vi "Fetch Rx Data (I16 multi).vi"(0 "Register Bus":T1, 2 "vertical range [Vpp]":dbl=2.0 format="%#_6p", 5 "number of samples":u32=8196, 9 "timeout [s]":dbl=10.0, 11 "error in":errorcluster, 13 "leading samples to trim":i32) -> (3 "scaling (V/code)":dbl, 4 "Register Bus (out)":T1, 6 "I":i16[](array[numeric]), 8 "Q":i16[](array[numeric]), 15 "error out":errorcluster)   [LabVIEW 2017]
doc: "Fetch Rx data from the device. It's required to call <b>Configure Stream</b> and <b>Initiate Stream</b> before calling this VI."
uses:
  <instrlib>/_niInstr/Register Bus/v0/Host/Public/Register Bus Session.ctl
  <instrlib>/_niInstr/Register Bus/v0/Host/Private/Session Data.ctl
  Rx FPGA VI Reference.ctl
  <vilib>/rvi/errors/niLvFpgaAdjustHostInterfaceError.vi
  <vilib>/rvi/interface/nirviMethod/nirviMethod.xnode
  <instrlib>/_niInstr/Register Bus/v0/Host/niInstr Register Bus v0 Host.lvlib
  <vilib>/FPGAPlugInAG/Dynamic/niLvFpga_ReadFifo_Dynamic.vi
  <vilib>/rvi/errors/niLvFpgaMergeErrorWithErrorCode.vi
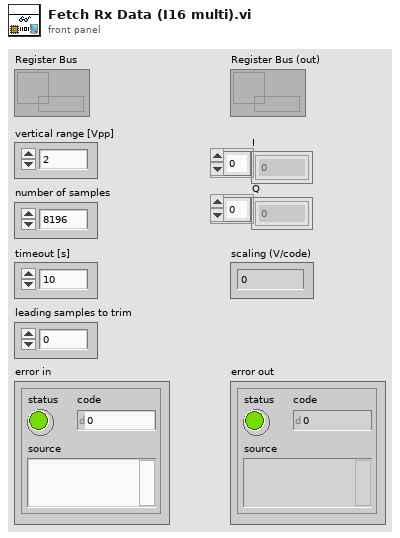
[diagram p1: front panel]
types:
  T1 = typedef "niInstr Register Bus v0 Host.lvlib/Register Bus Session.ctl" = refnum<queue>
  T2 = typedef "Rx FPGA VI Reference.ctl" = refnum<k20>
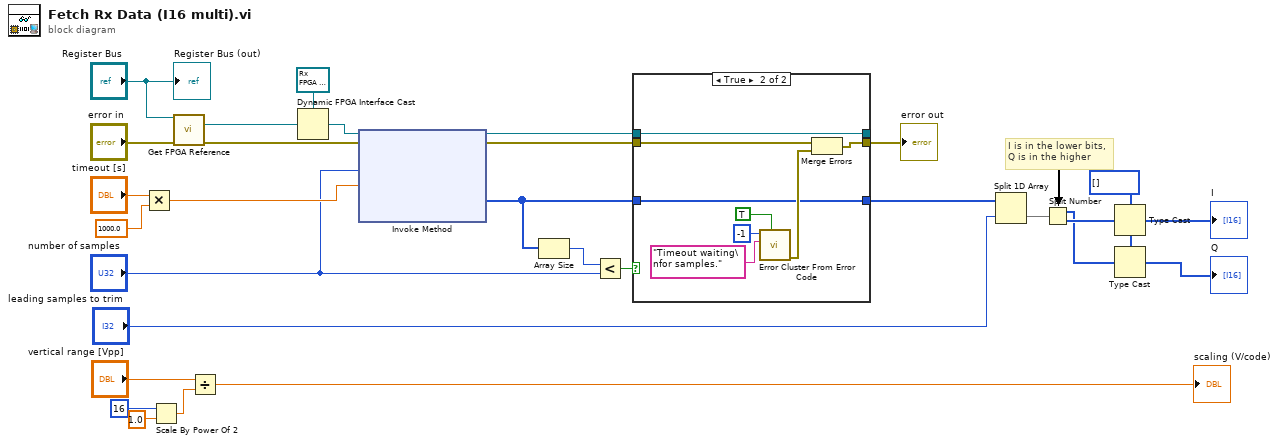
[diagram p0: block diagram]
diagram:
  w9 = i16[] []
  # "I is in the lower bits,\nQ is in the higher"
  n1 = Multiply(x="timeout [s]", y=1000.0) -> (x*y=w20:dbl)
  n2 = Scale By Power Of 2(n=i16 16 ("ADC Resolution (bits)"), x=1.0) -> (x*2^n=w12:dbl)
  n3 = call <instrlib>:"Get FPGA Reference.vi"("session in"="Register Bus", "error in"="error in") -> ("fpga ref"=w27:refnum<k20>, "error out"=w26:errorcluster)  [unwired: 11 in, 1 out]
  n4 = Divide(x="vertical range [Vpp]", y=w12) -> (x/y=→"scaling (V/code)":dbl)
  n5 = Dynamic FPGA Interface Cast(Session In=T2 refnum ("Type"), Type=w27) -> (Session Out=w25:T2)
  n6 = xnode "Invoke Method"("FPGA VI Reference In"=w25, "error in"=w26, "Number of Elements"="number of samples", "Timeout (ms)"=w20) -> ("FPGA VI Reference Out"=w23:T2, "error out"=w24:errorcluster, "Data"=w3:u32[])  [unwired: 1 out]
  n7 = Array Size(array=w3) -> (size(s)=w2:i32)
  n8 = Less?(x=w2, y="number of samples") -> (x < y?=w18:bool)
  n9 = case shown="True" w18 {
    tunnel: w23 -> [w32 w40]
    tunnel: w24 -> [w31 w37]
    tunnel: [w32 w40] -> _
    tunnel: [w31 w36] -> w16
    tunnel: [w30 w33] -> w1
    tunnel: w3 -> [w30 w33]
    frame False {
    }
    frame True {
      n10 = call <vilib>:"Error Cluster From Error Code.vi"("show call chain? (False)"=TRUE, "error message (\"\")"="Timeout waiting\nfor samples." ("error message (\"\")"), "error code (0)"=-1) -> ("error out"=w35:errorcluster)  [unwired: 6 in]
      n11 = Merge Errors(w37, w35) -> (w36:errorcluster)
    }
  }
  "error out" <- w16
  n12 = Split 1D Array(array=w1, index="leading samples to trim") -> (second subarray=w8:u32[])  [unwired: 1 out]
  n13 = Split Number(x=w8) -> (hi(x)=w4:u16[], lo(x)=w5:u16[])
  n14 = Type Cast(type=w9, x=w5) -> (*(type *) &x=→"I":i16[])
  n15 = Type Cast(type=w9, x=w4) -> (*(type *) &x=→"Q":i16[])
  "Register Bus (out)" <- "Register Bus"
